vi "Get subscription map.vi"(8 "error in (no error)":errorcluster {"code" format="Error %.0f"}, 11 "NATS Client in":refnum<class "NATS Client.lvclass">) -> (0 "error out":errorcluster {"code" format="Error %.0f"}, 2 "subscription map":refnum<data-value>, 3 "NATS Client out":refnum<class "NATS Client.lvclass">)   [LabVIEW 2020, in "NATS Client.lvlib" / "NATS Client.lvclass"]
uses:
  NATS Client.lvclass
  NATS Subscription/NATS Subscription.lvclass
  NATS Client.lvclass/NATS Client.ctl
  Subscription Map.ctl
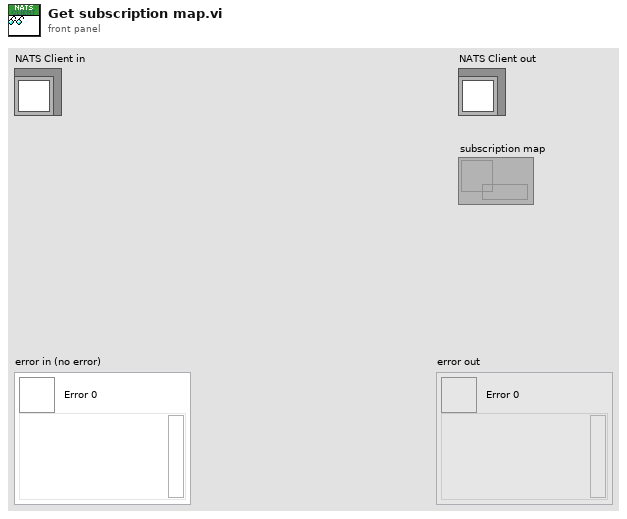
[diagram p1: front panel]
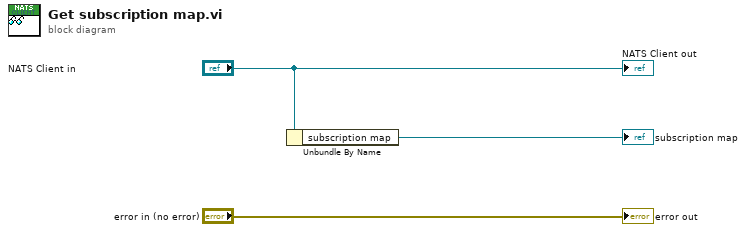
[diagram p0: block diagram]
diagram:
  n1 = Unbundle By Name("NATS Client in") -> ("subscription map"=→"subscription map":refnum<data-value>)
  "error out" <- "error in (no error)"
  "NATS Client out" <- "NATS Client in"
